vi "Set properties.vi"(8 "error in (no error)":errorcluster, 11 "Lockin SR830 in":refnum<class "Lockin SR830.lvclass">) -> (0 "error out":errorcluster, 3 "Lockin SR830 out":refnum<class "Lockin SR830.lvclass">)   [LabVIEW 2023, in "Lockin SR830.lvclass"]
uses:
  Lockin SR830.lvclass
  Lockin SR830.lvclass/Lockin SR830.ctl
  sr830/SR830.lvlib
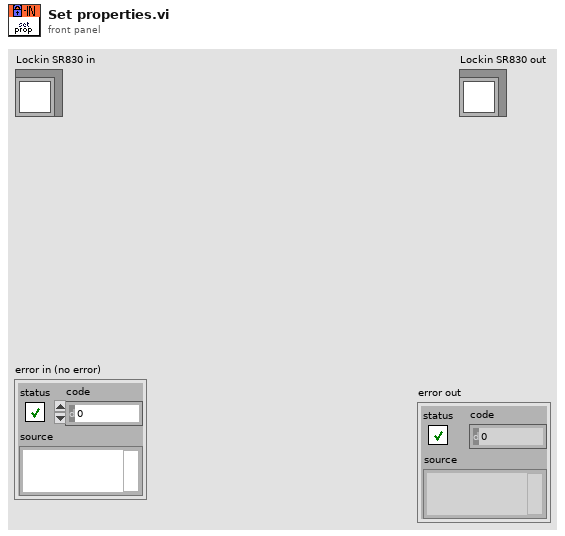
[diagram p1: front panel]
types:
  T1 = typedef "Lockin SR830.lvclass/Sensitivity.ctl" = u16
  T2 = typedef "SR830.lvlib/Tau.ctl" = u16
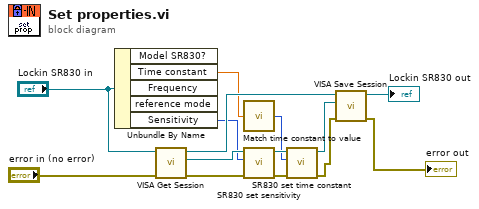
[diagram p0: block diagram]
diagram:
  n1 = Unbundle By Name("Lockin SR830 in") -> ("Time constant"=w5:dbl[unit], "Sensitivity"=w3:T1)  [unwired: 3 out]
  n2 = call-dynamic "VISA Get Session.vi"("error in (no error)"="error in (no error)", "Instrument.lvclass in"="Lockin SR830 in") -> ("error out"=w8:errorcluster, "VISA Resource Name"=w12:refnum<visa-resource-name>, "Instrument.lvclass out"=w14:refnum<class "Lockin SR830.lvclass">)  [unwired: 7 out]
  n3 = call "Match time constant to value.vi"("Time constant"=w5) -> ("Tau"=w4:T2)
  n4 = call "SR830 set sensitivity.vi"("error in (no error)"=w8, "Sensitivity"=w3, "VISA resource name"=w12) -> ("error out"=w7:errorcluster, "VISA resource name out"=w11:refnum<visa-resource-name>)  [unwired: 7 in]
  n5 = call "SR830 set time constant.vi"("error in (no error)"=w7, "Tau"=w4, "VISA resource name"=w11) -> ("error out"=w2:errorcluster, "VISA resource name out"=w10:refnum<visa-resource-name>)  [unwired: 7 in]
  n6 = call-dynamic "VISA Save Session.vi"("error in (no error)"=w2, "VISA Resource Name"=w10, "Instrument.lvclass in"=w14) -> ("error out"=→"error out":errorcluster, "Instrument.lvclass out"=→"Lockin SR830 out":refnum<class "Lockin SR830.lvclass">)  [unwired: 7 out]
